vi "CAN ID's.vi"() -> ()   [LabVIEW 2018]
panel:
  in  "CAN ID":T1={"RightMaster"=5, "RightSlaveA"=14, "RightSlaveB"=13, "LeftMaster"=1, "LeftSlaveA"=10, "LeftSlaveB"=12, "PCM"=0, "PDP"=0, "Intake"=11, "Pivot"=16, "Elevator"=4, "Right Climber"=2, "Left Climber"=3, "Shooter"=15}
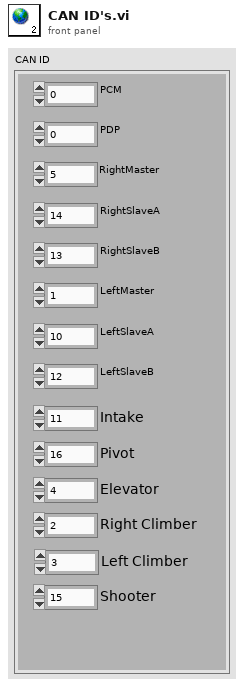
[diagram p1: front panel]
types:
  T1 = cluster{"RightMaster":u8, "RightSlaveA":u8, "RightSlaveB":u8, "LeftMaster":u8, "LeftSlaveA":u8, "LeftSlaveB":u8, "PCM":u8, "PDP":u8, "Intake":u8, "Pivot":u8, "Elevator":u8, "Right Climber":u8, "Left Climber":u8, "Shooter":u8}
diagram:
